vi "Edit Tree Items-Add Item to End.vi"(5 "Child Only?":bool, 6 "New Item Indentation":i32, 7 "Child Tag":string, 8 "error in (no error)":errorcluster, 9 "Child Text":string[](array[string]), 10 "Left Cell String":string, 11 "TreeControl in":refnum<class "TreeControl.lvclass">) -> (0 "error out":errorcluster, 2 "Edit Tree Items:Add Item to End":string, 3 "TreeControl out":refnum<class "TreeControl.lvclass">)   [LabVIEW 2015, in "TreeControl.lvclass"]
doc: "Adds an item after all existing items in the tree control.\n\nQControl Class wrapper around the <b>TreeControl : Edit Tree Items:Add Item to End Method</b>.\n<b> </b> <b> </b>\n©2016 Q Software Innovations, LLC (QSI)\nwritten by Quentin Alldredge\nproduced in LabVIEW 2015\n\nsupport@qsoftwareinnovations.com\nwww.qsoftwareinnovations.com\n\nAll rights reserved.\n\nRedistribution and use in source and binary forms, with or without modification, are permitted provided that the following conditions are met:\n\n * Redistributions of source code must retain the above copyright notice, this list of conditions and the following disclaimer.\n * Redistributions in binary form must reproduce the above copyright notice, this list of conditions and the following disclaimer in the documentation and/or other materials provided with the distribution.\n * Neither the name of Q Software Innovations, LLC. nor the names of its contributors may be used to endorse or promote products derived from this software without specific prior written permission.\n\nTHIS SOFTWARE IS PROVIDED BY THE COPYRIGHT HOLDERS AND CONTRIBUTORS \"AS IS\" AND ANY EXPRESS OR IMPLIED WARRANTIES, INCLUDING, BUT NOT LIMITED TO, THE IMPLIED WARRANTIES OF MERCHANTABILITY AND FITNESS FOR A PARTICULAR PURPOSE ARE DISCLAIMED. IN NO EVENT SHALL THE COPYRIGHT OWNER OR CONTRIBUTORS BE LIABLE FOR ANY DIRECT, INDIRECT, INCIDENTAL, SPECIAL, EXEMPLARY, OR CONSEQUENTIAL DAMAGES (INCLUDING, BUT NOT LIMITED TO, PROCUREMENT OF SUBSTITUTE GOODS OR SERVICES; LOSS OF USE, DATA, OR PROFITS; OR BUSINESS INTERRUPTION) HOWEVER CAUSED AND ON ANY THEORY OF LIABILITY, WHETHER IN CONTRACT, STRICT LIABILITY, OR TORT (INCLUDING NEGLIGENCE OR OTHERWISE) ARISING IN ANY WAY OUT OF THE USE OF THIS SOFTWARE, EVEN IF ADVISED OF THE POSSIBILITY OF SUCH DAMAGE."
uses:
  TreeControl.lvclass
  TreeControl.lvclass/TreeControl.ctl
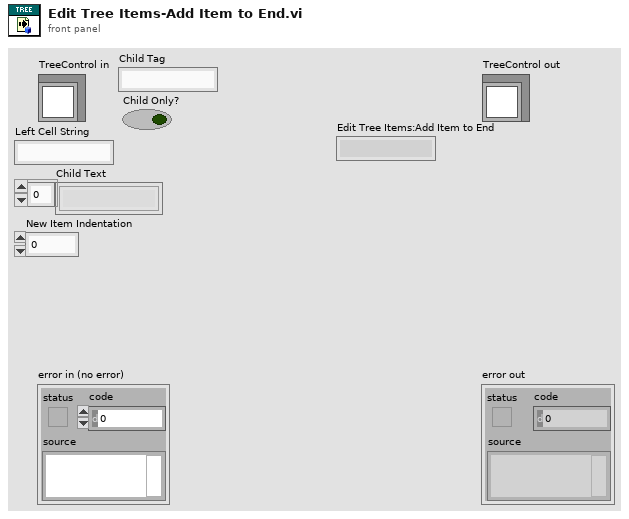
[diagram p1: front panel]
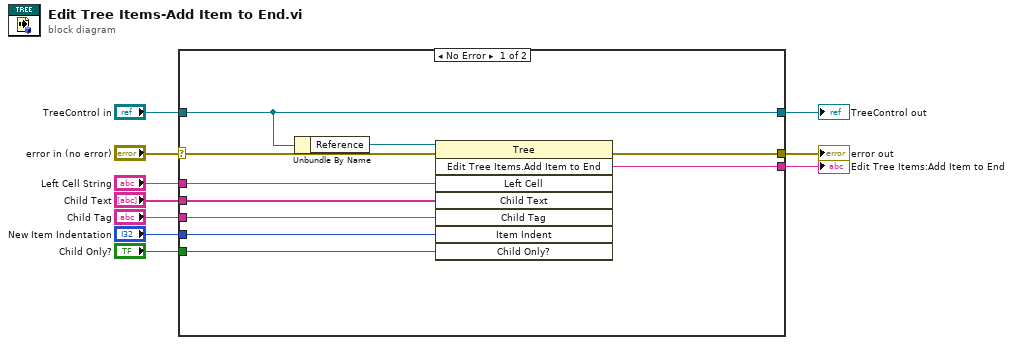
[diagram p0: block diagram]
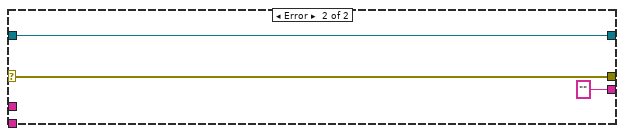
[diagram p2: hidden frame]
diagram:
  n1 = case shown="No Error" "error in (no error)" {
    selector: "error in (no error)" -> [w20 w23]
    tunnel: [w19 w23] -> w9
    tunnel: [w18 w22] -> w7
    tunnel: "TreeControl in" -> [w18 w22]
    tunnel: "Left Cell String" -> [w16 _]
    tunnel: [w15 "" ("Edit Tree Items:Add Item to End")] -> w5
    tunnel: "Child Text" -> [w14 _]
    tunnel: "Child Tag" -> [w13 _]
    tunnel: "New Item Indentation" -> [w12 _]
    tunnel: "Child Only?" -> [w11 _]
    frame No Error {
      n2 = Unbundle By Name(w18) -> ("Reference"=w17:refnum<vi>)
      n3 = invoke class="Tree" method="Edit Tree Items.Add Item to End"(reference=w17, error in=w20, "Left Cell"=w16, "Child Text"=w14, "Child Tag"=w13, "Item Indent"=w12, "Child Only?"=w11) -> (error out=w19:errorcluster, "Edit Tree Items:Add Item to End"=w15:string)  [unwired: 1 in, 6 out]
    }
    frame Error {
    }
  }
  "error out" <- w9
  "TreeControl out" <- w7
  "Edit Tree Items:Add Item to End" <- w5
